vi "PLC_comm.vi"() -> ()   [LabVIEW 2017]
uses:
  <vilib>/addons/database/NI_Database_API.lvlib
  <vilib>/NI/Modbus Library/API/Wrapper/API Main.lvlib
  <vilib>/NI/Modbus Library/API/Wrapper/Create TCP Master.vi
  <vilib>/NI/Modbus Library/API/Master/Modbus Master.lvclass
  Global/DATA LOG.vi
  Global/Global 1.vi
  <vilib>/DATA AHEAD/SP7/typedefs/PLC Type.ctl
  <vilib>/DATA AHEAD/SP7/SP7.lvlib
  <vilib>/DATA AHEAD/SP7/functions/write/write bool array.vi
  <vilib>/DATA AHEAD/SP7/functions/read/read bool array.vi
  <vilib>/DATA AHEAD/SP7/functions/read/read int array.vi
  <vilib>/DATA AHEAD/SP7/functions/read/read String.vi
  <userlib>/_OpenG.lib/comparison/comparison.llb/String Changed__ogtk.vi
  <vilib>/addons/database/Connection.llb/DB Tools Open Connec (String).vi
panel:
  in  "timeout [ms]":i32=5000
  in  "String":string
  out "Array":u16[](array[numeric])
  out "element":u16
  out "length 2":i32
  out "substring":string
  out "length":i32
  out "reversed":string
  out "PLC 4":bool
  out "PLC 3":bool
  out "PLC 2":bool
  out "PLC 1":bool
  out "IP1 4":string
  out "IP1 3":string
  out "IP1 2":string
  out "IP1":string
  out "register values 4":u16[](array[numeric])
  out "ASCII VALUE 4":string[](array[string])
  out "BARCODE  4":string
  out "register values 3":u16[](array[numeric])
  out "ASCII VALUE 3":string[](array[string])
  out "BARCODE  3":string
  in  "stop":bool
  out "error out":errorcluster
  in  "error in (no error)":errorcluster
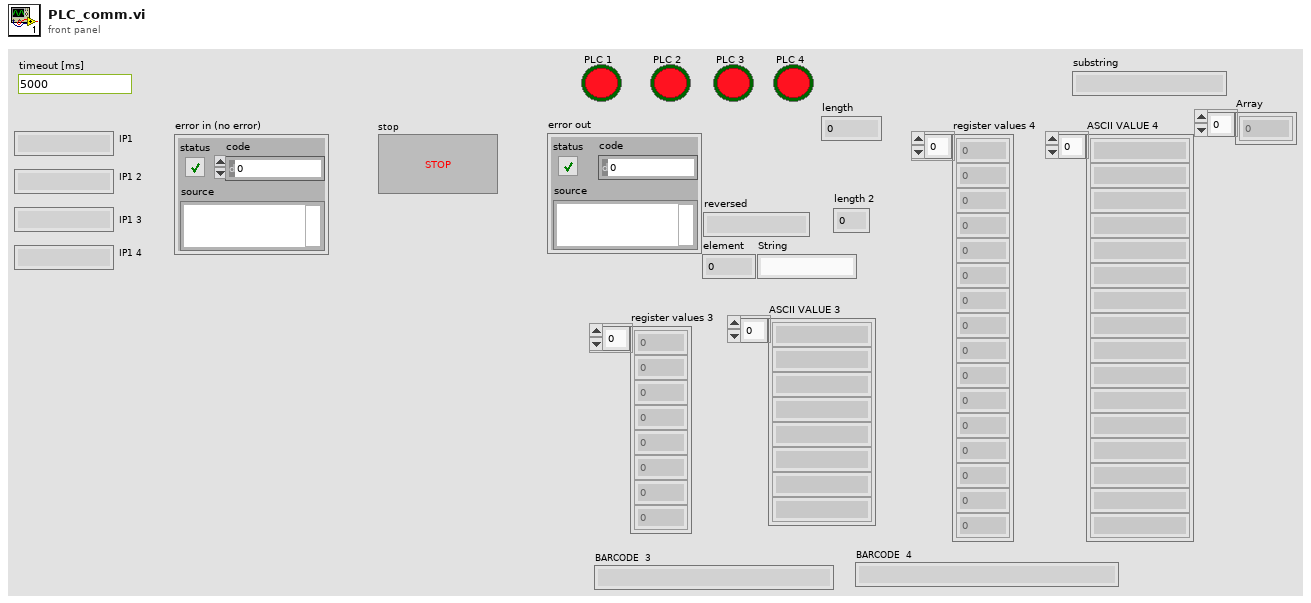
[diagram p1: front panel]
types:
  T1 = typedef "SP7.lvlib/PLC Type.ctl" = enum16{"S7 200", "S7 300/400", "S7 1200", "S7 1500", "LOGO!8"}
  T2 = typedef "NI_Database_API.lvlib/Conn ObjectReference.ctl" = refnum<k1>
  T3 = typedef "SP7.lvlib/S7 Connection.ctl" = cluster{"TCP Connection Ref":refnum<k5>, "IP address":string, "timeout ms":i32, "Connected?":bool, "PLC Type":T1, "Rack S7 400":u8, "Slot S7 400":u8, "PDU Size":u16, "connection semaphore":T4}
  T4 = typedef "Semaphore RefNum" = refnum<k1>
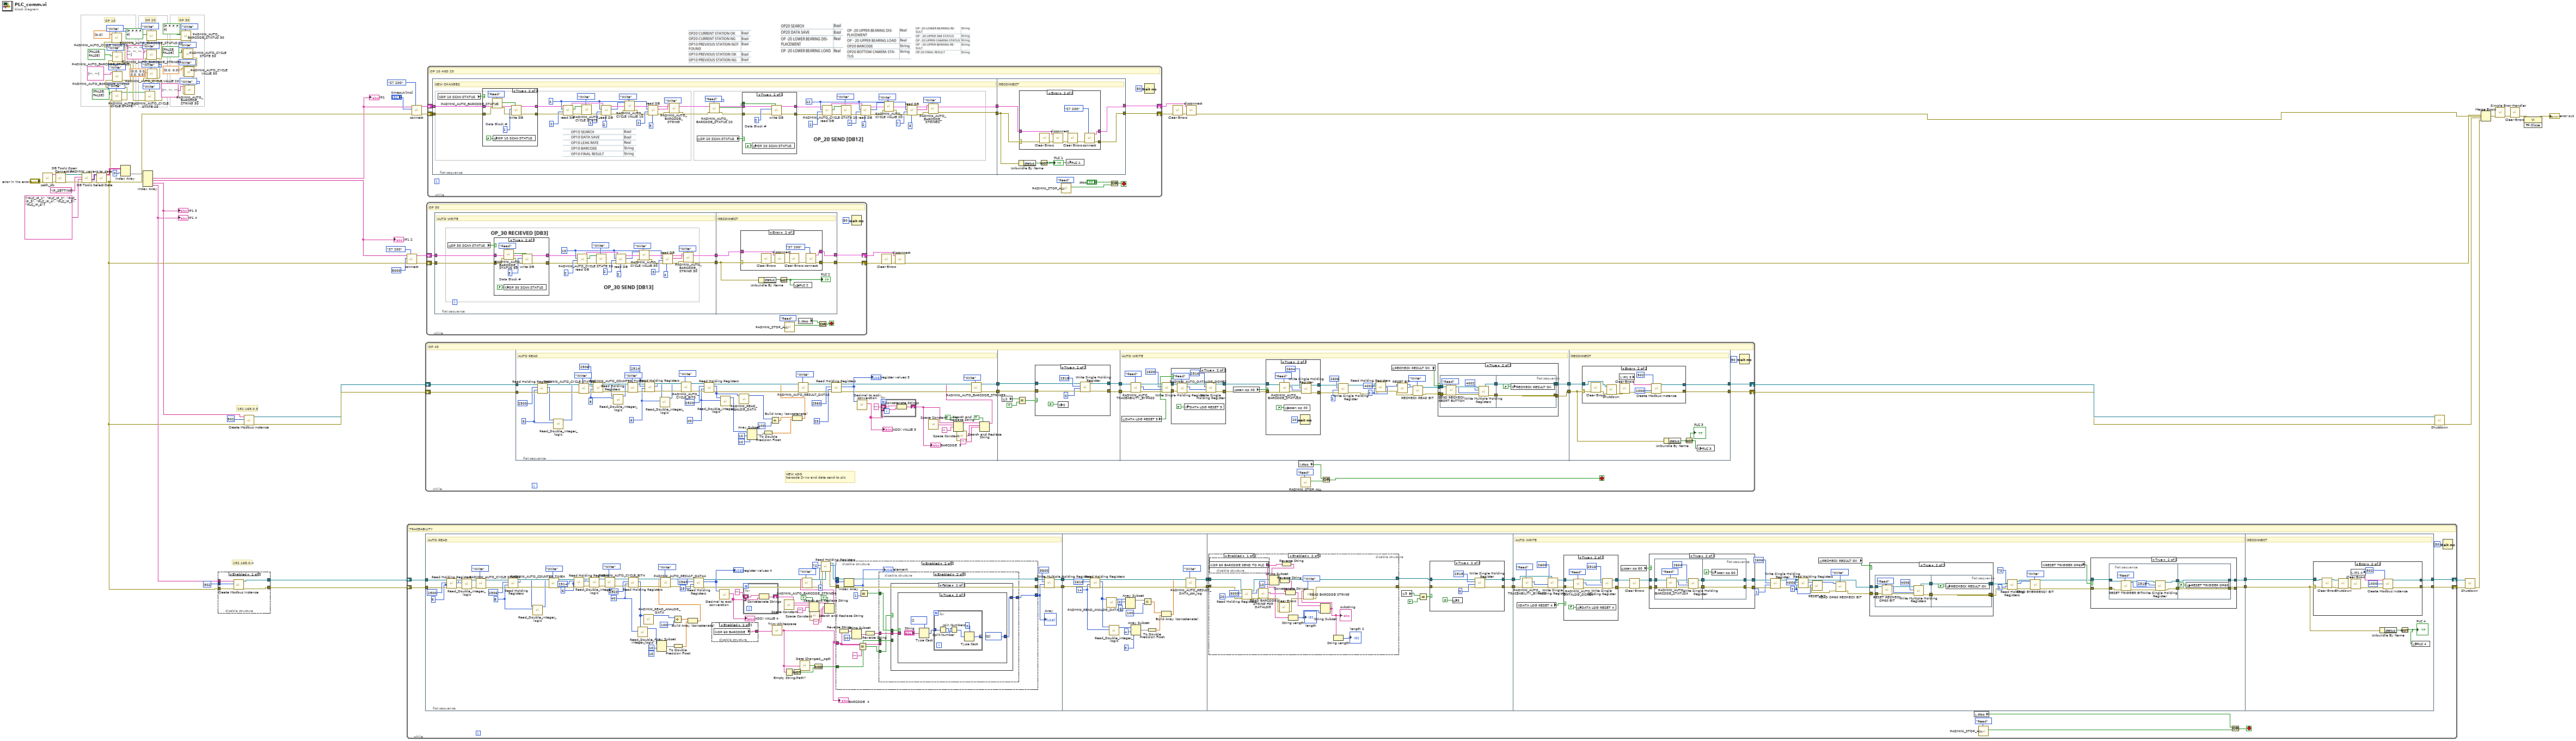
[diagram p0: block diagram]
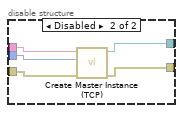
[diagram p2: hidden frame]
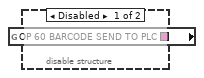
[diagram p3: hidden frame]
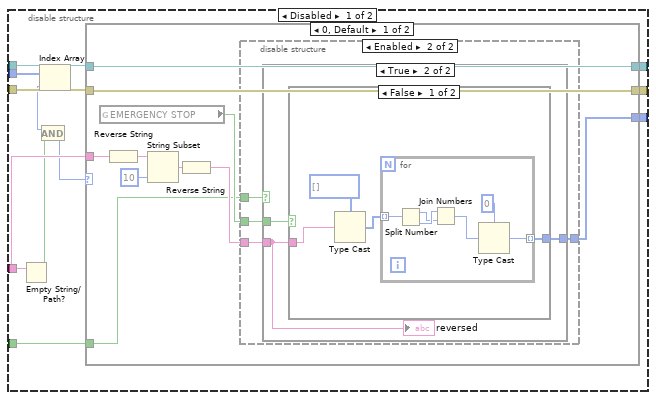
[diagram p4: hidden frame]
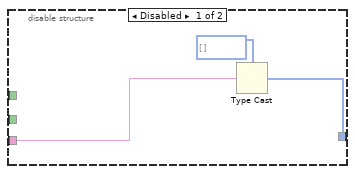
[diagram p5: hidden frame]
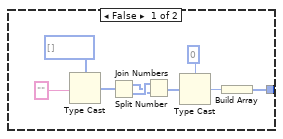
[diagram p6: hidden frame]
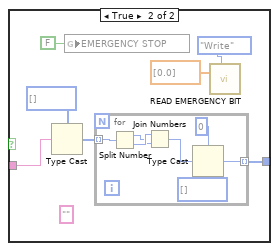
[diagram p7: hidden frame]
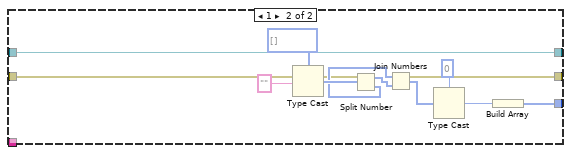
[diagram p8: hidden frame]
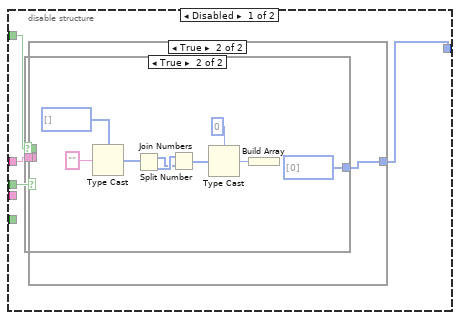
[diagram p9: hidden frame]
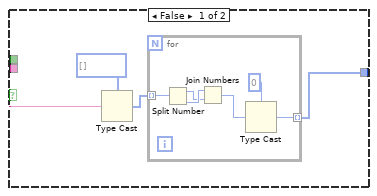
[diagram p10: hidden frame]
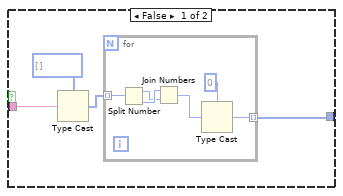
[diagram p11: hidden frame]
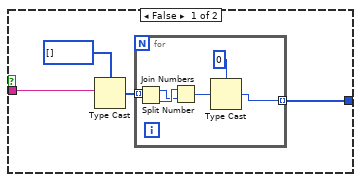
[diagram p12: hidden frame]
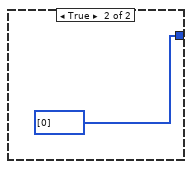
[diagram p13: hidden frame]
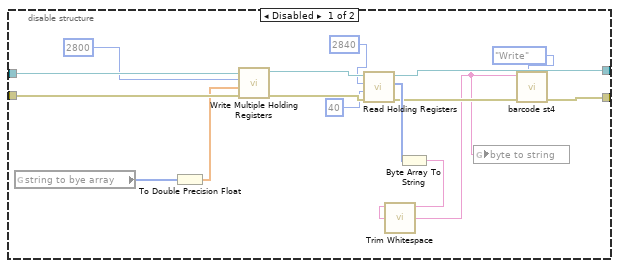
[diagram p14: hidden frame]
diagram:
  w31 = bool[] [FALSE, FALSE] ("Input")
  # "OP 30"
  # "OP 20"
  # "OP 10"
  # "192.168.0.3"
  # "192.168.0.4"
  n1 = call "path_db.vi"("error in"="error in (no error)") -> ("error out"=w78:errorcluster, "resulting string"=w83:string)  [unwired: 9 in]
  n2 = call-poly <vilib>:"DB Tools Open Connection.vi"("error in (no error)"=w78, "connection information"=w83) -> ("error out"=w82:errorcluster, "connection reference"=w81:T2)  [unwired: 6 in]
  n3 = call <vilib>:"DB Tools Select Data.vi"("error in (no error)"=w82, "columns"=string[] ["PLC_IP_1", "PLC_IP_2", "PLC_IP_3", "PLC_IP_4", "PLC_IP_5", "PLC_IP_6"], "table"="IP_SETTING", "connection reference"=w81) -> ("error out"=w80:errorcluster, "data"=w79:variant[][])  [unwired: 2 in, 1 out]
  n4 = call "PADMINI_varient_to_data.vi"("error in (no error)"=w80, "data"=w79) -> ("error out"=w46:errorcluster, "Array"=w74:string[][])  [unwired: 8 in]
  n5 = call "PADMINI_AUTO_CYCLE STATE.vi"("Enum"=enum16{"Read", "Write"}."Write", "error in (no error)"=w46, "Input"=w31) -> ("error out"=w44:errorcluster)  [unwired: 7 in, 1 out]
  n6 = call "PADMINI_AUTO_BARCODE_STRING.vi"("Enum"=enum16{"Read", "Write"}."Write", "error in (no error)"=w44, "Input"=string[] ["", ""]) -> ("error out"=w40:errorcluster)  [unwired: 7 in, 1 out]
  n7 = call "PADMINI_AUTO_BARCODE_STATUS.vi"("Enum"=enum16{"Read", "Write"}."Write", "error in (no error)"=w40, "I/P"=bool[] [FALSE, FALSE]) -> ("error out"=w38:errorcluster)  [unwired: 7 in, 1 out]
  n8 = call "PADMINI_AUTO_CYCLE VALUE 10.vi"("Enum"=enum16{"Read", "Write"}."Write", "error in (no error)"=w38, "Input"=dbl[] [0.0]) -> ("error out"=w32:errorcluster)  [unwired: 7 in, 1 out]
  n9 = Index Array(array=w74, index (row)=0) -> (element=w73:string[])  [unwired: 1 in]
  n10 = Index Array(array=w73) -> (element #1=w50:string, element #2=w17:string, element #3=w68:string, element #4=w67:string)  [unwired: 4 in]
  "IP1" <- w50
  "IP1 2" <- w17
  "IP1 3" <- w68
  "IP1 4" <- w67
  n11 = call "PADMINI_AUTO_CYCLE STATE 20.vi"("Enum"=enum16{"Read", "Write"}."Write", "error in (no error)"=w32, "Input"=w31) -> ("error out"=w29:errorcluster)  [unwired: 7 in, 1 out]
  n12 = call "PADMINI_AUTO_CYCLE VALUE 20.vi"("Enum"=enum16{"Read", "Write"}."Write", "error in (no error)"=w29, "Input"=dbl[] [0.0, 0.0, 0.0, 0.0]) -> ("error out"=w25:errorcluster)  [unwired: 7 in, 1 out]
  n13 = call "PADMINI_AUTO_BARCODE_STRING2.vi"("Enum"=enum16{"Read", "Write"}."Write", "error in (no error)"=w25, "Input"=string[] ["", "", "", "", "", "", ""]) -> ("error out"=w22:errorcluster)  [unwired: 7 in, 1 out]
  n14 = call "PADMINI_AUTO_BARCODE_STATUS 20.vi"("Enum"=enum16{"Read", "Write"}."Write", "error in (no error)"=w22, "I/P"=bool[] [FALSE, FALSE, FALSE, FALSE, FALSE]) -> ("error out"=w14:errorcluster)  [unwired: 7 in, 1 out]
  n15 = call "PADMINI_AUTO_BARCODE_STATUS 30.vi"("Enum"=enum16{"Read", "Write"}."Write", "error in (no error)"=w14, "I/P"=bool[] [FALSE, FALSE, FALSE, FALSE, FALSE]) -> ("error out"=w11:errorcluster)  [unwired: 7 in, 1 out]
  n16 = call "PADMINI_AUTO_CYCLE STATE 30.vi"("Enum"=enum16{"Read", "Write"}."Write", "error in (no error)"=w11, "Input"=bool[] [FALSE, FALSE]) -> ("error out"=w10:errorcluster)  [unwired: 7 in, 1 out]
  n17 = call "PADMINI_AUTO_CYCLE VALUE 30.vi"("Enum"=enum16{"Read", "Write"}."Write", "error in (no error)"=w10, "Input"=dbl[] [0.0, 0.0]) -> ("error out"=w6:errorcluster)  [unwired: 7 in, 1 out]
  n18 = call "PADMINI_AUTO_BARCODE_STRING 30.vi"("Enum"=enum16{"Read", "Write"}."Write", "error in (no error)"=w6, "Input"=string[] ["", "", ""]) -> ()  [unwired: 7 in, 2 out]
  n19 = disable-structure shown="Enabled" {
    disable-tunnel: w67 -> [w88 w92]
    disable-tunnel: u16 502 ("port (502)") -> [w87 w91]
    disable-tunnel: [w86 w90] -> w61
    disable-tunnel: [w85 w89] -> w60
    disable-tunnel: w46 -> [w84 w93]
    frame Enabled {
      n20 = call-poly <vilib>:"Create Modbus Instance.vi"("error in"=w84, "port (502)"=w87, "address"=w88) -> ("error out"=w85:errorcluster, "TCP master instance"=w86:refnum<class "Modbus Master.lvclass">)  [unwired: 7 in]
    }
    frame Disabled {
      n21 = call <vilib>:"Create Master Instance (TCP).vi"("error in (no error)"=w93, "port (502)"=w91, "address"=w92) -> ("error out"=w89:errorcluster, "TCP master instance"=w90:refnum<class "Modbus Master.lvclass">)  [unwired: 7 in]
    }
  }
  n22 = call-poly <vilib>:"Create Modbus Instance.vi"("error in"=w46, "port (502)"=u16 502, "address"=w68) -> ("error out"=w63:errorcluster, "TCP master instance"=w62:refnum<class "Modbus Master.lvclass">)  [unwired: 7 in]
  n23 = call <vilib>:"connect.vi"("PLC Type"=PLC_Type."S7 200" ("PLC Type 2"), "error in (no error)"=w46, "timeout [ms]"=5000 ("timeout [ms] 2"), "IP address"=w17) -> ("error out"=w19:errorcluster, "S7 Connection out"=w18:T3)  [unwired: 6 in]
  n24 = while {
    shift-right: [w108] -> w54
    shift-left: w61 -> [w110]
    shift-right: [w107] -> w55
    shift-left: w60 -> [w109]
    stop <- w101 stop-if-true
    # "TRACEABILITY"
    n25 = flat-sequence {
      tunnel: w110 -> [w183]
      tunnel: w109 -> [w182]
      tunnel: [w123] -> w100
      tunnel: [w126] -> w99
      tunnel: w100 -> [w352]
      tunnel: [w350] -> w98
      tunnel: w99 -> [w351]
      tunnel: [w348] -> w97
      tunnel: w98 -> [w370]
      tunnel: w97 -> [w368]
      tunnel: [w373] -> w96
      tunnel: [w372] -> w95
      tunnel: [w426] -> w105
      tunnel: w96 -> [w449]
      tunnel: w95 -> [w448]
      tunnel: [w424] -> w94
      tunnel: [w531] -> w107
      tunnel: [w533] -> w108
      tunnel: w105 -> [w534]
      tunnel: w94 -> [w529]
      frame #0 {
        (unwired) 10 ("length")
        w145 = u16 40 ("number of inputs")
        w147 = u16 6 ("number of inputs")
        w150 = u16 8 ("number of inputs")
        w153 = u16 6 ("number of inputs")
        # "AUTO READ"
        n26 = call-dynamic "Read Holding Registers.vi"("error in"=w182, "number of inputs"=w153, "starting address"=u16 2500, "Modbus master in"=w183) -> ("error out"=w175:errorcluster, "register values"=w154:u16[], "Modbus master out"=w174:refnum<class "Modbus Master.lvclass">)  [unwired: 5 in]
        n27 = call "Read_Double_integer_logic.vi"("Numeric"=w153, "register values"=w154) -> ("Array"=w152:u16[])  [unwired: 9 in]
        n28 = call "PADMINI_AUTO_CYCLE STATE4.vi"("Enum"=enum16{"Read", "Write"}."Write", "error in (no error)"=w175, "Input"=w152) -> ("error out"=w167:errorcluster)  [unwired: 7 in, 1 out]
        n29 = call-dynamic "Read Holding Registers.vi"("error in"=w167, "number of inputs"=w150, "starting address"=u16 2506, "Modbus master in"=w174) -> ("error out"=w173:errorcluster, "register values"=w151:u16[], "Modbus master out"=w172:refnum<class "Modbus Master.lvclass">)  [unwired: 5 in]
        n30 = call "Read_Double_integer_logic.vi"("Numeric"=w150, "register values"=w151) -> ("Array"=w149:u16[])  [unwired: 9 in]
        n31 = call "PADMINI_AUTO_COUNTER_TIME4.vi"("Enum"=enum16{"Read", "Write"}."Write", "error in (no error)"=w173, "Input"=w149) -> ("error out"=w165:errorcluster)  [unwired: 7 in, 1 out]
        n32 = call-dynamic "Read Holding Registers.vi"("error in"=w165, "number of inputs"=w147, "starting address"=u16 2514, "Modbus master in"=w172) -> ("error out"=w171:errorcluster, "register values"=w148:u16[], "Modbus master out"=w170:refnum<class "Modbus Master.lvclass">)  [unwired: 5 in]
        n33 = call "Read_Double_integer_logic.vi"("Numeric"=w147, "register values"=w148) -> ("Array"=w146:u16[])  [unwired: 9 in]
        n34 = call "PADMINI_AUTO_CYCLE_BIT4.vi"("Enum"=enum16{"Read", "Write"}."Write", "error in (no error)"=w171, "Input"=w146) -> ("error out"=w163:errorcluster)  [unwired: 7 in, 1 out]
        n35 = call-dynamic "Read Holding Registers.vi"("error in"=w163, "number of inputs"=w145, "starting address"=u16 2520, "Modbus master in"=w170) -> ("error out"=w169:errorcluster, "register values"=w142:u16[], "Modbus master out"=w168:refnum<class "Modbus Master.lvclass">)  [unwired: 5 in]
        n36 = call "Read_Double_integer_logic.vi"("Numeric"=w145, "register values"=w142) -> ("Array"=w144:u16[])  [unwired: 9 in]
        n37 = call "PADMINI_READ_ANALOG_DATA.vi"("register values"=w142) -> ("Array"=w141:i32[])  [unwired: 10 in]
        n38 = Array Subset(array=w144, index=10) -> (w157:u16[])  [unwired: 1 in]
        n39 = Divide(x=w141, y=u16 100 ("number of inputs")) -> (x/y=w155:dbl[])
        n40 = To Double Precision Float(number=w157) -> (double precision float=w156:dbl[])
        n41 = Build Array (concatenate)(w155, w156) -> (w143:dbl[])
        n42 = call "PADMINI_AUTO_RESULT_DATA4.vi"("Enum"=enum16{"Read", "Write"}."Write", "error in (no error)"=w169, "Input"=w143) -> ("error out"=w161:errorcluster)  [unwired: 7 in, 1 out]
        n43 = call-dynamic "Read Holding Registers.vi"("error in"=w161, "number of inputs"=u16 25, "starting address"=u16 2560, "Modbus master in"=w168) -> ("error out"=w121:errorcluster, "register values"=w176:u16[], "Modbus master out"=w119:refnum<class "Modbus Master.lvclass">)  [unwired: 5 in]
        "register values 4" <- w176
        n44 = disable-structure shown="Enabled" {
          disable-tunnel: [w187 w188] -> w120
          frame Disabled {
            n45 = global read "Global 1.vi" "OP 60 BARCODE SEND TO PLC"() -> (w187:string)
          }
          frame Enabled {
            n46 = global read "Global 1.vi" "OP 60 BARCODE"() -> (w188:string)
          }
        }
        n47 = call "Decimal to ascii converstion.vi"("DECIMAL VALUE"=w176) -> ("array w/ subset deleted"=w185:string[])  [unwired: 9 in]
        "ASCII VALUE 4" <- w185
        n48 = for {
          tunnel: w185 -> [w345] mode=indexing
          shift-right: [w344] -> w132
          shift-left: "" -> [w343]
          n49 = Concatenate Strings(w343, w345) -> (w344:string)
        }
        n50 = call <vilib>:"Trim Whitespace.vi"("string"=w120) -> ("trimmed string"=w111:string)  [unwired: 1 in]
        "BARCODE  4" <- w111
        n51 = call <vilib>:"Space Constant.vi"() -> ("String"=w140:string)
        n52 = Empty String/Path?(string/path=w111) -> (empty?=w129:bool)
        n53 = Not(x=w129) -> (.not. x?=w130:bool)
        n54 = call-poly <userlib>:"Data Changed__ogtk.vi"("String"=w111) -> ("Changed"=w128:bool)
        n55 = Search and Replace String(replace all?=TRUE ("replace all? (F)"), input string=w132, search string=w140, replace string="") -> (result string=w135:string)  [unwired: 4 in, 3 out]
        n56 = call <vilib>:"Space Constant.vi"() -> ("String"=w136:string)
        n57 = And(x=w128, y=w130) -> (x .and. y?=w112:bool)
        n58 = Search and Replace String(replace all?=TRUE ("replace all? (F)"), input string=w135, search string=w136, replace string="") -> (result string=w131:string)  [unwired: 4 in, 3 out]
        n59 = call "PADMINI_AUTO_BARCODE_STRING4.vi"("Enum"=enum16{"Read", "Write"}."Write", "error in (no error)"=w121, "Input"=w131) -> ("error out"=w118:errorcluster)  [unwired: 7 in, 1 out]
        n60 = call-dynamic "Read Holding Registers.vi"("error in"=w118, "number of inputs"=u16 3, "starting address"=u16 72, "Modbus master in"=w119) -> ("error out"=w116:errorcluster, "register values"=w113:u16[], "Modbus master out"=w117:refnum<class "Modbus Master.lvclass">)  [unwired: 5 in]
        n61 = disable-structure shown="Enabled" {
          disable-tunnel: w111 -> [w199 w265]
          disable-tunnel: w112 -> [w198 w274]
          disable-tunnel: [w197 w275] -> w127
          disable-tunnel: [w196 w276] -> w125
          disable-tunnel: [w195 w277] -> w124
          disable-tunnel: w117 -> [w194 w277]
          disable-tunnel: w116 -> [w193 w276]
          disable-tunnel: w113 -> [w192 w272]
          frame Disabled {
            n62 = Empty String/Path?(string/path=w199) -> (empty?=w190:bool)
            n63 = Index Array(array=w192) -> (element=w191:u16)  [unwired: 1 in]
            n64 = And(x=w191, y=w190) -> (x .and. y?=w189:u16)
            n65 = case shown="0, Default" w189 {
              tunnel: w194 -> [w201 w254]
              tunnel: [w201 w254] -> w195
              tunnel: w193 -> [w200 w253]
              tunnel: [w200 w253] -> w196
              tunnel: w199 -> [w205 _]
              tunnel: w198 -> [w203 _]
              tunnel: [w202 w252] -> w197
              frame 0, Default {
                n66 = global read "Global 1.vi" "EMERGENCY STOP"() -> (w204:bool)
                n67 = Reverse String(1:w205) -> (0:w209:string)
                n68 = String Subset(string=w209, length (rest)=10 ("length (rest)")) -> (substring=w207:string)  [unwired: 1 in]
                n69 = Reverse String(1:w207) -> (0:w206:string)
                n70 = disable-structure shown="Enabled" {
                  disable-tunnel: w206 -> [w212 w215]
                  disable-tunnel: [w211 w213] -> w202
                  disable-tunnel: w204 -> [_ w216]
                  disable-tunnel: w203 -> [_ w214]
                  frame Disabled {
                    n71 = Type Cast(type=u16[] [], x=w212) -> (*(type *) &x=w211:u16[])
                  }
                  frame Enabled {
                    n72 = case shown="True" w214 {
                      tunnel: w216 -> [_ w227]
                      tunnel: w215 -> [_ w226]
                      tunnel: [w217 w228] -> w213
                      frame False {
                        n73 = Type Cast(type=u16[] [], x="") -> (*(type *) &x=w224:u16[])
                        n74 = Split Number(x=w224) -> (hi(x)=w221:u8[], lo(x)=w222:u8[])
                        n75 = Join Numbers(hi=w222, lo=w221) -> ((hi.lo)=w220:u16[])
                        n76 = Type Cast(type=u16 0, x=w220) -> (*(type *) &x=w218:u16)
                        n77 = Build Array(w218) -> (w217:u16[])
                      }
                      frame True {
                        n78 = case shown="False" w227 {
                          tunnel: w226 -> [w230 w239]
                          tunnel: [w229 w242] -> w228
                          frame False {
                            n79 = Type Cast(type=u16[] [], x=w230) -> (*(type *) &x=w231:u16[])
                            n80 = for {
                              tunnel: w231 -> [w238] mode=indexing
                              tunnel: [w234] -> w229 mode=indexing
                              n81 = Split Number(x=w238) -> (hi(x)=w236:u8, lo(x)=w237:u8)
                              n82 = Join Numbers(hi=w237, lo=w236) -> ((hi.lo)=w235:u16)
                              n83 = Type Cast(type=u16 0, x=w235) -> (*(type *) &x=w234:u16)
                            }
                          }
                          frame True {
                            (unwired) ""
                            (unwired) u16[] []
                            n84 = Type Cast(type=u16[] [], x=w239) -> (*(type *) &x=w243:u16[])
                            n85 = global write "Global 1.vi" "EMERGENCY STOP"(FALSE ("EMERGENCY STOP")) -> ()
                            n86 = for {
                              tunnel: w243 -> [w251] mode=indexing
                              tunnel: [w247] -> w242 mode=indexing
                              n87 = Split Number(x=w251) -> (hi(x)=w249:u8, lo(x)=w250:u8)
                              n88 = Join Numbers(hi=w250, lo=w249) -> ((hi.lo)=w248:u16)
                              n89 = Type Cast(type=u16 0, x=w248) -> (*(type *) &x=w247:u16)
                            }
                            n90 = call "READ EMERGENCY BIT.vi"("Enum"=enum16{"Read", "Write"}."Write", "Array In"=dbl[] [0.0]) -> ()  [unwired: 8 in, 2 out]
                          }
                        }
                        "reversed" <- w226
                      }
                    }
                  }
                }
              }
              frame 1 {
                n91 = Type Cast(type=u16[] [], x="") -> (*(type *) &x=w261:u16[])
                n92 = Split Number(x=w261) -> (hi(x)=w258:u8[], lo(x)=w259:u8[])
                n93 = Join Numbers(hi=w259, lo=w258) -> ((hi.lo)=w257:u16[])
                n94 = Type Cast(type=u16 0, x=w257) -> (*(type *) &x=w255:u16)
                n95 = Build Array(w255) -> (w252:u16[])
              }
            }
          }
          frame Enabled {
            n96 = Reverse String(1:w265) -> (0:w270:string)
            n97 = Index Array(array=w272) -> (element=w273:u16)  [unwired: 1 in]
            "element" <- w273
            n98 = String Subset(string=w270, length (rest)=10 ("length (rest)")) -> (substring=w269:string)  [unwired: 1 in]
            n99 = Equal?(x=w265, y="") -> (x = y?=w263:bool)
            n100 = Equal?(x=w273, y=u16 1 ("x")) -> (x = y?=w266:bool)
            n101 = Reverse String(1:w269) -> (0:w267:string)
            n102 = disable-structure shown="Enabled" {
              disable-tunnel: [w281 w317] -> w275
              disable-tunnel: w274 -> [w280 w314]
              disable-tunnel: w266 -> [w279 w316]
              disable-tunnel: w267 -> [w278 w318]
              disable-tunnel: w265 -> [_ _]
              disable-tunnel: w263 -> [_ w315]
              frame Disabled {
                n103 = case shown="True" w280 {
                  tunnel: w278 -> [w283 w294]
                  tunnel: [w282 w293] -> w281
                  tunnel: w279 -> [_ w292]
                  frame False {
                    n104 = Type Cast(type=u16[] [], x=w283) -> (*(type *) &x=w284:u16[])
                    n105 = for {
                      tunnel: w284 -> [w291] mode=indexing
                      tunnel: [w287] -> w282 mode=indexing
                      n106 = Split Number(x=w291) -> (hi(x)=w289:u8, lo(x)=w290:u8)
                      n107 = Join Numbers(hi=w290, lo=w289) -> ((hi.lo)=w288:u16)
                      n108 = Type Cast(type=u16 0, x=w288) -> (*(type *) &x=w287:u16)
                    }
                  }
                  frame True {
                    n109 = case shown="True" w292 {
                      tunnel: w294 -> [w296 _]
                      tunnel: [w295 u16[] [0]] -> w293
                      frame False {
                        n110 = Type Cast(type=u16[] [], x=w296) -> (*(type *) &x=w297:u16[])
                        n111 = for {
                          tunnel: w297 -> [w304] mode=indexing
                          tunnel: [w300] -> w295 mode=indexing
                          n112 = Split Number(x=w304) -> (hi(x)=w302:u8, lo(x)=w303:u8)
                          n113 = Join Numbers(hi=w303, lo=w302) -> ((hi.lo)=w301:u16)
                          n114 = Type Cast(type=u16 0, x=w301) -> (*(type *) &x=w300:u16)
                        }
                      }
                      frame True {
                        n115 = Type Cast(type=u16[] [], x="" ("OP 60 BARCODE SEND TO PLC")) -> (*(type *) &x=w312:u16[])
                        n116 = Split Number(x=w312) -> (hi(x)=w309:u8[], lo(x)=w310:u8[])
                        n117 = Join Numbers(hi=w310, lo=w309) -> ((hi.lo)=w308:u16[])
                        n118 = Type Cast(type=u16 0, x=w308) -> (*(type *) &x=w306:u16)
                        n119 = Build Array(w306) -> ()  [unwired: 1 out]
                      }
                    }
                  }
                }
              }
              frame Enabled {
                n120 = case shown="False" w315 {
                  tunnel: w318 -> [w321 _]
                  tunnel: [w320 u16[] [0]] -> w317
                  tunnel: w316 -> [w319 _]
                  tunnel: w314 -> [_ _]
                  frame False {
                    n121 = case shown="True" w319 {
                      tunnel: w321 -> [w323 _]
                      tunnel: [w322 u16[] [0]] -> w320
                      frame False {
                        n122 = Type Cast(type=u16[] [], x=w323) -> (*(type *) &x=w324:u16[])
                        n123 = for {
                          tunnel: w324 -> [w331] mode=indexing
                          tunnel: [w326] -> w322 mode=indexing
                          n124 = Split Number(x=w331) -> (hi(x)=w329:u8, lo(x)=w330:u8)
                          n125 = Join Numbers(hi=w330, lo=w329) -> ((hi.lo)=w328:u16)
                          n126 = Type Cast(type=u16 0, x=w328) -> (*(type *) &x=w326:u16)
                        }
                      }
                      frame True {
                        n127 = Type Cast(type=u16[] [], x="String") -> (*(type *) &x=w334:u16[])
                        n128 = for {
                          tunnel: w334 -> [w341] mode=indexing
                          tunnel: [w337] -> _ mode=indexing
                          n129 = Split Number(x=w341) -> (hi(x)=w339:u8, lo(x)=w340:u8)
                          n130 = Join Numbers(hi=w340, lo=w339) -> ((hi.lo)=w338:u16)
                          n131 = Type Cast(type=u16 0, x=w338) -> (*(type *) &x=w337:u16)
                        }
                      }
                    }
                  }
                  frame True {
                  }
                }
              }
            }
          }
        }
        "Array" <- w127
        n132 = call-dynamic "Write Multiple Holding Registers.vi"("error in"=w125, "registers to write"=w127, "starting address"=u16 3600, "Modbus master in"=w124) -> ("error out"=w126:errorcluster, "Modbus master out"=w123:refnum<class "Modbus Master.lvclass">)  [unwired: 6 in]
      }
      frame #1 {
        w361 = u16 14 ("number of inputs")
        n133 = call-dynamic "Read Holding Registers.vi"("error in"=w351, "number of inputs"=w361, "starting address"=u16 2610, "Modbus master in"=w352) -> ("error out"=w349:errorcluster, "register values"=w359:u16[], "Modbus master out"=w350:refnum<class "Modbus Master.lvclass">)  [unwired: 5 in]
        n134 = call "PADMINI_READ_ANALOG_DATA 2y.vi"("register values"=w359) -> ("Array"=w354:i32[])  [unwired: 10 in]
        n135 = call "Read_Double_integer_logic.vi"("Numeric"=w361, "register values"=w359) -> ("Array"=w360:u16[])  [unwired: 9 in]
        n136 = Array Subset(array=w354, index=0, length=4) -> (w353:i32[])
        n137 = Array Subset(array=w360, index=4, length=3) -> (w364:u16[])
        n138 = Divide(x=w353, y=u16 100 ("number of inputs")) -> (x/y=w362:dbl[])
        n139 = To Double Precision Float(number=w364) -> (double precision float=w363:dbl[])
        n140 = Build Array (concatenate)(w362, w363) -> (w347:dbl[])
        n141 = call "PADMINI_AUTO_RESULT_DATA_st4_log.vi"("Enum"=enum16{"Read", "Write"}."Write", "error in (no error)"=w349, "Input"=w347) -> ("error out"=w348:errorcluster)  [unwired: 7 in, 1 out]
      }
      frame #2 {
        n142 = disable-structure shown="Enabled" {
          disable-tunnel: w370 -> [w390 w411]
          disable-tunnel: [w389 w410] -> w369
          disable-tunnel: w368 -> [w388 w409]
          disable-tunnel: [w387 w404] -> w367
          frame Disabled {
            n143 = global read "DATA LOG.vi" "string to bye array"() -> (w377:u8[])
            n144 = To Double Precision Float(number=w377) -> (double precision float=w376:dbl[])
            n145 = call-dynamic "Write Multiple Holding Registers.vi"("error in"=w388, "registers to write"=w376, "starting address"=u16 2800, "Modbus master in"=w390) -> ("error out"=w384:errorcluster, "Modbus master out"=w385:refnum<class "Modbus Master.lvclass">)  [unwired: 6 in]
            n146 = call-dynamic "Read Holding Registers.vi"("error in"=w384, "number of inputs"=u16 40 ("starting address"), "starting address"=u16 2840, "Modbus master in"=w385) -> ("error out"=w379:errorcluster, "register values"=w382:u16[], "Modbus master out"=w389:refnum<class "Modbus Master.lvclass">)  [unwired: 5 in]
            n147 = Byte Array To String(unsigned byte array=w382) -> (string=w378:string)
            n148 = call <vilib>:"Trim Whitespace.vi"("string"=w378) -> ()  [unwired: 1 in, 1 out]
            n149 = global write "DATA LOG.vi" "byte to string"(w378) -> ()
            n150 = call "barcode st4.vi"("Enum"=enum16{"Read", "Write"}."Write", "error in (no error)"=w379, "Input"=w378) -> ("error out"=w387:errorcluster)  [unwired: 7 in, 1 out]
          }
          frame Enabled {
            n151 = disable-structure shown="Enabled" {
              disable-tunnel: [w412 _] -> w397
              frame Enabled {
                n152 = global read "Global 1.vi" "OP 60 BARCODE SEND TO PLC"() -> (w412:string)
              }
              frame Disabled {
              }
            }
            n153 = call-dynamic "Read Holding Registers.vi"("error in"=w409, "number of inputs"=u16 20, "starting address"=u16 6000, "Modbus master in"=w411) -> ("error out"=w406:errorcluster, "register values"=w405:u16[], "Modbus master out"=w410:refnum<class "Modbus Master.lvclass">)  [unwired: 5 in]
            n154 = call "READ BARCODE STRING FOR DATALOG.vi"("error in (no error)"=w406, "DECIMAL VALUE"=w405) -> ("error out"=w392:errorcluster, "String"=w402:string)  [unwired: 7 in, 1 out]
            n155 = call <vilib>:"Clear Errors.vi"("error in (no error)"=w392) -> ("error out"=w391:errorcluster)  [unwired: 5 in, 1 out]
            n156 = Reverse String(1:w397) -> (0:w401:string)
            n157 = String Subset(string=w401, offset (0)=10) -> (substring=w399:string)  [unwired: 1 in]
            n158 = Reverse String(1:w399) -> (0:w398:string)
            n159 = Concatenate Strings(w398, w402) -> (w396:string)
            n160 = String Length(string=w397) -> (length=w395:i32)
            "length" <- w395
            n161 = String Subset(string=w396, length (rest)=w395) -> (substring=w393:string)  [unwired: 1 in]
            "substring" <- w393
            n162 = call "REAS BARCODE STRING.vi"("error in (no error)"=w391, "Input"=w393, "Enum"=enum16{"Read", "Write"}."Write") -> ("error out"=w404:errorcluster)  [unwired: 7 in, 1 out]
            n163 = String Length(string=w393) -> (length=→"length 2":i32)
          }
        }
        n164 = global read "DATA LOG.vi" "3"() -> (w375:bool)
        n165 = Equal?(x=w375, y=TRUE) -> (x = y?=w371:bool)
        n166 = case shown="True" w371 {
          tunnel: [w414 w419] -> w373
          tunnel: [w413 w418] -> w372
          tunnel: w369 -> [w414 w416]
          tunnel: w367 -> [w413 w415]
          frame False {
          }
          frame True {
            n167 = global write "DATA LOG.vi" "3"(FALSE) -> ()
            n168 = call-dynamic "Write Single Holding Register.vi"("error in"=w415, "register to write"=u16 0 ("address"), "address"=u16 2518, "Modbus master in"=w416) -> ("error out"=w418:errorcluster, "Modbus master out"=w419:refnum<class "Modbus Master.lvclass">)  [unwired: 6 in]
          }
        }
      }
      frame #3 {
        w443 = u16 2 ("number of inputs")
        # "AUTO WRITE"
        n169 = global read "DATA LOG.vi" "DATA LOG RESET 4"() -> (w452:bool)
        n170 = call "PADMINI_AUTO_TRACEABILITY_BYPASS.vi"("Enum"=enum16{"Read", "Write"}."Read", "error in (no error)"=w448) -> ("error out"=w460:errorcluster, "O/P"=w458:u16)  [unwired: 8 in]
        n171 = call-dynamic "Write Single Holding Register.vi"("error in"=w460, "register to write"=w458, "address"=u16 2600, "Modbus master in"=w449) -> ("error out"=w456:errorcluster, "Modbus master out"=w453:refnum<class "Modbus Master.lvclass">)  [unwired: 6 in]
        n172 = case shown="True" w452 {
          tunnel: w456 -> [w518 w528]
          tunnel: [w519 w527] -> w454
          tunnel: w453 -> [w519 w526]
          tunnel: [w518 w521] -> w423
          frame False {
          }
          frame True {
            n173 = call "PADMINI_AUTO_DATALOG_DONE4.vi"("Enum"=enum16{"Read", "Write"}."Read", "error in (no error)"=w528) -> ("error out"=w525:errorcluster, "O/P"=w522:u16)  [unwired: 8 in]
            n174 = global write "DATA LOG.vi" "DATA LOG RESET 4"(FALSE ("DATA LOG RESET 4")) -> ()
            n175 = call-dynamic "Write Single Holding Register.vi"("error in"=w525, "register to write"=w522, "address"=u16 2516, "Modbus master in"=w526) -> ("error out"=w521:errorcluster, "Modbus master out"=w527:refnum<class "Modbus Master.lvclass">)  [unwired: 6 in]
          }
        }
        n176 = global read "DATA LOG.vi" "scan op 60"() -> (w446:bool)
        n177 = call <vilib>:"Clear Errors.vi"("error in (no error)"=w423) -> ("error out"=w422:errorcluster)  [unwired: 5 in, 1 out]
        n178 = case shown="True" w446 {
          tunnel: [w500 w506] -> w455
          tunnel: w454 -> [w500 w505]
          tunnel: w422 -> [w499 w504]
          tunnel: [w499 w503] -> w451
          frame False {
          }
          frame True {
            n179 = flat-sequence {
              tunnel: w505 -> [w513]
              tunnel: w504 -> [w511]
              tunnel: [w514] -> w502
              tunnel: [w507] -> w501
              tunnel: [w516] -> w503
              tunnel: [w517] -> w506
              tunnel: w502 -> [w517]
              tunnel: w501 -> [w516]
              frame #0 {
                n180 = call "PADMINI_AUTO_BARCODE_STATUS4.vi"("Enum"=enum16{"Read", "Write"}."Read", "error in (no error)"=w511) -> ("error out"=w510:errorcluster, "O/P"=w509:u16)  [unwired: 8 in]
                n181 = call-dynamic "Write Single Holding Register.vi"("error in"=w510, "register to write"=w509, "address"=u16 2604, "Modbus master in"=w513) -> ("error out"=w507:errorcluster, "Modbus master out"=w514:refnum<class "Modbus Master.lvclass">)  [unwired: 6 in]
              }
              frame #1 {
                n182 = global write "DATA LOG.vi" "scan op 60"(FALSE ("scan op 60")) -> ()
              }
            }
          }
        }
        n183 = call-dynamic "Write Single Holding Register.vi"("error in"=w451, "register to write"=u16 1 ("address"), "address"=u16 2606, "Modbus master in"=w455) -> ("error out"=w440:errorcluster, "Modbus master out"=w437:refnum<class "Modbus Master.lvclass">)  [unwired: 6 in]
        n184 = call-dynamic "Read Holding Registers.vi"("error in"=w440, "number of inputs"=w443, "starting address"=u16 4006, "Modbus master in"=w437) -> ("error out"=w445:errorcluster, "register values"=w444:u16[])  [unwired: 5 in, 1 out]
        n185 = call "RESET BIT.vi"("Numeric"=w443, "register values"=w444) -> ("Array"=w439:u16[])  [unwired: 9 in]
        n186 = global read "Global 1.vi" "RECHECK RESULT OK"() -> (w438:bool)
        n187 = call "READ OP60 RECHECK BIT.vi"("Enum"=enum16{"Read", "Write"}."Write", "error in (no error)"=w445, "Input"=w439) -> ("error out"=w436:errorcluster)  [unwired: 7 in, 1 out]
        n188 = case shown="True" w438 {
          tunnel: w437 -> [w481 w482]
          tunnel: [w481 w487] -> w434
          tunnel: w436 -> [w480 w486]
          tunnel: [w480 w485] -> w431
          frame False {
          }
          frame True {
            n189 = flat-sequence {
              tunnel: w486 -> [w490]
              tunnel: [w494] -> w484
              tunnel: [w489] -> w483
              tunnel: w482 -> [w488]
              tunnel: [w497] -> w485
              tunnel: [w498] -> w487
              tunnel: w484 -> [w498]
              tunnel: w483 -> [w497]
              frame #0 {
                n190 = call "RESET RECHECK OP60 BIT.vi"("Enum"=enum16{"Read", "Write"}."Read", "error in (no error)"=w490) -> ("error out"=w491:errorcluster, "Array 2"=w493:u16[])  [unwired: 8 in]
                n191 = call-dynamic "Write Multiple Holding Registers.vi"("error in"=w491, "registers to write"=w493, "starting address"=u16 4006, "Modbus master in"=w488) -> ("error out"=w489:errorcluster, "Modbus master out"=w494:refnum<class "Modbus Master.lvclass">)  [unwired: 6 in]
              }
              frame #1 {
                n192 = global write "Global 1.vi" "RECHECK RESULT OK"(FALSE ("RECHECK RESULT OK")) -> ()
              }
            }
          }
        }
        n193 = call-dynamic "Read Holding Registers.vi"("error in"=w431, "number of inputs"=u16 1, "starting address"=u16 70 ("address"), "Modbus master in"=w434) -> ("error out"=w430:errorcluster, "register values"=w429:u16[], "Modbus master out"=w427:refnum<class "Modbus Master.lvclass">)  [unwired: 5 in]
        n194 = call "READ EMERGENCY BIT.vi"("Enum"=enum16{"Read", "Write"}."Write", "error in (no error)"=w430, "Array In"=w429) -> ("error out"=w425:errorcluster)  [unwired: 7 in, 1 out]
        n195 = global read "Global 1.vi" "RESET TRIGGER OP60"() -> (w428:bool)
        n196 = case shown="True" w428 {
          tunnel: w427 -> [w462 w468]
          tunnel: w425 -> [w461 w467]
          tunnel: [w462 w466] -> w426
          tunnel: [w461 w464] -> w424
          frame False {
          }
          frame True {
            n197 = flat-sequence {
              tunnel: w468 -> [w476]
              tunnel: w467 -> [w472]
              tunnel: [w475] -> w465
              tunnel: [w474] -> w463
              tunnel: [w479] -> w466
              tunnel: w465 -> [w479]
              tunnel: [w478] -> w464
              tunnel: w463 -> [w478]
              frame #0 {
                n198 = call "RESET TRIGGER BIT.vi"("Enum"=enum16{"Read", "Write"}."Read", "error in (no error)"=w472) -> ("error out"=w471:errorcluster, "Numeric 2"=w469:u16)  [unwired: 8 in]
                n199 = call-dynamic "Write Single Holding Register.vi"("error in"=w471, "register to write"=w469, "address"=u16 2518 ("starting address"), "Modbus master in"=w476) -> ("error out"=w474:errorcluster, "Modbus master out"=w475:refnum<class "Modbus Master.lvclass">)  [unwired: 6 in]
              }
              frame #1 {
                n200 = global write "Global 1.vi" "RESET TRIGGER OP60"(FALSE ("RESET TRIGGER OP60")) -> ()
              }
            }
          }
        }
      }
      frame #4 {
        # "RECONNECT"
        n201 = case shown="Error" w529 {
          selector: w529 -> [w535 w545]
          tunnel: [w536 w542] -> w533
          tunnel: w534 -> [w536 w540]
          tunnel: [w535 w541] -> w531
          frame No Error {
          }
          frame Error {
            n202 = call <vilib>:"Clear Errors.vi"("error in (no error)"=w545) -> ("error out"=w539:errorcluster)  [unwired: 5 in, 1 out]
            n203 = call-dynamic "Shutdown.vi"("error in"=w539, "Modbus master in"=w540) -> ("error out"=w538:errorcluster)  [unwired: 9 in]
            n204 = local read "IP1 4"() -> (w543:string)
            n205 = call <vilib>:"Clear Errors.vi"("error in (no error)"=w538) -> ("error out"=w544:errorcluster)  [unwired: 5 in, 1 out]
            n206 = call-poly <vilib>:"Create Modbus Instance.vi"("error in"=w544, "connect timeout ms"=1000, "port (502)"=u16 502, "address"=w543) -> ("error out"=w541:errorcluster, "TCP master instance"=w542:refnum<class "Modbus Master.lvclass">)  [unwired: 6 in]
          }
        }
        n207 = Unbundle By Name(w529) -> ("status"=w532:bool)
        n208 = Not(x=w532) -> (.not. x?=w530:bool)
        "PLC 4" <- w530
        n209 = global write "Global 1.vi" "PLC 4"(w530) -> ()
      }
    }
    n210 = local read "stop"() -> (w102:bool)
    n211 = call "PADMINI_STOP_ALL.vi"("Enum"=enum16{"Read", "Write"}."Read") -> ("Boolean 2"=w103:bool)  [unwired: 9 in, 1 out]
    n212 = Or(x=w102, y=w103) -> (x .or. y?=w101:bool)
    n213 = Wait (ms)(milliseconds to wait=u32 50) -> ()  [unwired: 1 out]
  }
  n214 = call <vilib>:"connect.vi"("PLC Type"=PLC_Type."S7 200" ("PLC Type 2"), "error in (no error)"=w46, "timeout [ms]"="timeout [ms]", "IP address"=w50) -> ("error out"=w49:errorcluster, "S7 Connection out"=w48:T3)  [unwired: 6 in]
  n215 = while {
    shift-right: [w559] -> w58
    shift-left: w62 -> [w561]
    shift-right: [w558] -> w57
    shift-left: w63 -> [w560]
    stop <- w551 stop-if-true
    # "NEW ADD\nbarcode Sr no and date send to plc"
    # "OP 40"
    n216 = flat-sequence {
      tunnel: w561 -> [w618]
      tunnel: w560 -> [w617]
      tunnel: [w603] -> w550
      tunnel: [w594] -> w548
      tunnel: w550 -> [w628]
      tunnel: [w629] -> w549
      tunnel: w548 -> [w627]
      tunnel: [w626] -> w547
      tunnel: w549 -> [w665]
      tunnel: [w644] -> w556
      tunnel: [w642] -> w555
      tunnel: w547 -> [w669]
      tunnel: [w714] -> w558
      tunnel: [w717] -> w559
      tunnel: w556 -> [w716]
      tunnel: w555 -> [w712]
      frame #0 {
        w581 = u16 40 ("number of inputs")
        w585 = u16 6 ("number of inputs")
        w588 = u16 8 ("number of inputs")
        w589 = u16 6 ("number of inputs")
        # "AUTO READ"
        n217 = call-dynamic "Read Holding Registers.vi"("error in"=w617, "number of inputs"=w589, "starting address"=u16 2500, "Modbus master in"=w618) -> ("error out"=w611:errorcluster, "register values"=w592:u16[], "Modbus master out"=w610:refnum<class "Modbus Master.lvclass">)  [unwired: 5 in]
        n218 = call "Read_Double_integer_logic.vi"("Numeric"=w589, "register values"=w592) -> ("Array"=w590:u16[])  [unwired: 9 in]
        n219 = call "PADMINI_AUTO_CYCLE STATE3.vi"("Enum"=enum16{"Read", "Write"}."Write", "error in (no error)"=w611, "Input"=w590) -> ("error out"=w602:errorcluster)  [unwired: 7 in, 1 out]
        n220 = call-dynamic "Read Holding Registers.vi"("error in"=w602, "number of inputs"=w588, "starting address"=u16 2506, "Modbus master in"=w610) -> ("error out"=w609:errorcluster, "register values"=w587:u16[], "Modbus master out"=w608:refnum<class "Modbus Master.lvclass">)  [unwired: 5 in]
        n221 = call "Read_Double_integer_logic.vi"("Numeric"=w588, "register values"=w587) -> ("Array"=w586:u16[])  [unwired: 9 in]
        n222 = call "PADMINI_AUTO_COUNTER_TIME3.vi"("Enum"=enum16{"Read", "Write"}."Write", "error in (no error)"=w609, "Input"=w586) -> ("error out"=w600:errorcluster)  [unwired: 7 in, 1 out]
        n223 = call-dynamic "Read Holding Registers.vi"("error in"=w600, "number of inputs"=w585, "starting address"=u16 2514, "Modbus master in"=w608) -> ("error out"=w607:errorcluster, "register values"=w584:u16[], "Modbus master out"=w606:refnum<class "Modbus Master.lvclass">)  [unwired: 5 in]
        n224 = call "Read_Double_integer_logic.vi"("Numeric"=w585, "register values"=w584) -> ("Array"=w583:u16[])  [unwired: 9 in]
        n225 = call "PADMINI_AUTO_CYCLE_BIT3.vi"("Enum"=enum16{"Read", "Write"}."Write", "error in (no error)"=w607, "Input"=w583) -> ("error out"=w598:errorcluster)  [unwired: 7 in, 1 out]
        n226 = call-dynamic "Read Holding Registers.vi"("error in"=w598, "number of inputs"=w581, "starting address"=u16 2520, "Modbus master in"=w606) -> ("error out"=w605:errorcluster, "register values"=w572:u16[], "Modbus master out"=w582:refnum<class "Modbus Master.lvclass">)  [unwired: 5 in]
        n227 = call "Read_Double_integer_logic.vi"("Numeric"=w581, "register values"=w572) -> ("Array"=w577:u16[])  [unwired: 9 in]
        n228 = call "PADMINI_READ_ANALOG_DATA.vi"("register values"=w572) -> ("Array"=w571:i32[])  [unwired: 10 in]
        n229 = Array Subset(array=w577, index=10, length=10) -> (w576:u16[])
        n230 = To Double Precision Float(number=w576) -> (double precision float=w575:dbl[])
        n231 = Divide(x=w571, y=u16 100 ("number of inputs")) -> (x/y=w574:dbl[])
        n232 = Build Array (concatenate)(w574, w575) -> (w573:dbl[])
        n233 = call "PADMINI_AUTO_RESULT_DATA3.vi"("Enum"=enum16{"Read", "Write"}."Write", "error in (no error)"=w605, "Input"=w573) -> ("error out"=w596:errorcluster)  [unwired: 7 in, 1 out]
        n234 = call-dynamic "Read Holding Registers.vi"("error in"=w596, "number of inputs"=u16 25, "starting address"=u16 2560, "Modbus master in"=w582) -> ("error out"=w604:errorcluster, "register values"=w612:u16[], "Modbus master out"=w603:refnum<class "Modbus Master.lvclass">)  [unwired: 5 in]
        "register values 3" <- w612
        n235 = call "Decimal to ascii converstion.vi"("DECIMAL VALUE"=w612) -> ("array w/ subset deleted"=w620:string[])  [unwired: 9 in]
        "ASCII VALUE 3" <- w620
        n236 = for {
          tunnel: w620 -> [w624] mode=indexing
          shift-right: [w623] -> w563
          shift-left: "" -> [w622]
          n237 = Concatenate Strings(w622, w624) -> (w623:string)
        }
        "BARCODE  3" <- w563
        n238 = call <vilib>:"Space Constant.vi"() -> ("String"=w570:string)
        n239 = Search and Replace String(replace all?=TRUE ("replace all? (F)"), input string=w563, search string=w570, replace string="") -> (result string=w565:string)  [unwired: 4 in, 3 out]
        n240 = call <vilib>:"Space Constant.vi"() -> ("String"=w566:string)
        n241 = Search and Replace String(replace all?=TRUE ("replace all? (F)"), input string=w565, search string=w566, replace string="") -> (result string=w562:string)  [unwired: 4 in, 3 out]
        n242 = call "PADMINI_AUTO_BARCODE_STRING3.vi"("Enum"=enum16{"Read", "Write"}."Write", "error in (no error)"=w604, "Input"=w562) -> ("error out"=w594:errorcluster)  [unwired: 7 in, 1 out]
      }
      frame #1 {
        n243 = global read "DATA LOG.vi" "2"() -> (w630:bool)
        n244 = Equal?(x=w630, y=TRUE) -> (x = y?=w625:bool)
        n245 = case shown="True" w625 {
          tunnel: w628 -> [w632 w638]
          tunnel: w627 -> [w633 w636]
          tunnel: [w632 w637] -> w629
          tunnel: [w633 w635] -> w626
          frame False {
          }
          frame True {
            n246 = global write "DATA LOG.vi" "2"(FALSE) -> ()
            n247 = call-dynamic "Write Single Holding Register.vi"("error in"=w636, "register to write"=u16 0 ("address"), "address"=u16 2518, "Modbus master in"=w638) -> ("error out"=w635:errorcluster, "Modbus master out"=w637:refnum<class "Modbus Master.lvclass">)  [unwired: 6 in]
          }
        }
      }
      frame #2 {
        w651 = u16 2 ("number of inputs")
        # "AUTO WRITE"
        n248 = global read "DATA LOG.vi" "DATA LOG RESET 3"() -> (w657:bool)
        n249 = call "PADMINI_AUTO_TRACEABILITY_BYPASS.vi"("Enum"=enum16{"Read", "Write"}."Read", "error in (no error)"=w669) -> ("error out"=w668:errorcluster, "O/P"=w666:u16)  [unwired: 8 in]
        n250 = call-dynamic "Write Single Holding Register.vi"("error in"=w668, "register to write"=w666, "address"=u16 2600, "Modbus master in"=w665) -> ("error out"=w663:errorcluster, "Modbus master out"=w660:refnum<class "Modbus Master.lvclass">)  [unwired: 6 in]
        n251 = case shown="True" w657 {
          tunnel: w663 -> [w702 w711]
          tunnel: [w701 w710] -> w661
          tunnel: w660 -> [w701 w709]
          tunnel: [w702 w704] -> w658
          frame False {
          }
          frame True {
            n252 = call "PADMINI_AUTO_DATALOG_DONE3.vi"("Enum"=enum16{"Read", "Write"}."Read", "error in (no error)"=w711) -> ("error out"=w708:errorcluster, "O/P"=w705:u16)  [unwired: 8 in]
            n253 = global write "DATA LOG.vi" "DATA LOG RESET 3"(FALSE ("DATA LOG RESET 3")) -> ()
            n254 = call-dynamic "Write Single Holding Register.vi"("error in"=w708, "register to write"=w705, "address"=u16 2516, "Modbus master in"=w709) -> ("error out"=w704:errorcluster, "Modbus master out"=w710:refnum<class "Modbus Master.lvclass">)  [unwired: 6 in]
          }
        }
        n255 = global read "DATA LOG.vi" "scan op 40"() -> (w654:bool)
        n256 = case shown="True" w654 {
          tunnel: [w690 w700] -> w662
          tunnel: w661 -> [w690 w699]
          tunnel: w658 -> [w689 w698]
          tunnel: [w689 w697] -> w656
          frame False {
          }
          frame True {
            n257 = call "PADMINI_AUTO_BARCODE_STATUS3.vi"("Enum"=enum16{"Read", "Write"}."Read", "error in (no error)"=w698) -> ("error out"=w695:errorcluster, "O/P"=w694:u16)  [unwired: 8 in]
            n258 = global write "DATA LOG.vi" "scan op 40"(FALSE ("scan op 40")) -> ()
            n259 = Wait (ms)(milliseconds to wait=u32 20) -> ()  [unwired: 1 out]
            n260 = call-dynamic "Write Single Holding Register.vi"("error in"=w695, "register to write"=w694, "address"=u16 2604, "Modbus master in"=w699) -> ("error out"=w697:errorcluster, "Modbus master out"=w700:refnum<class "Modbus Master.lvclass">)  [unwired: 6 in]
          }
        }
        n261 = call-dynamic "Write Single Holding Register.vi"("error in"=w656, "register to write"=u16 1 ("address"), "address"=u16 2606, "Modbus master in"=w662) -> ("error out"=w646:errorcluster, "Modbus master out"=w648:refnum<class "Modbus Master.lvclass">)  [unwired: 6 in]
        n262 = call-dynamic "Read Holding Registers.vi"("error in"=w646, "number of inputs"=w651, "starting address"=u16 4002, "Modbus master in"=w648) -> ("error out"=w647:errorcluster, "register values"=w653:u16[], "Modbus master out"=w645:refnum<class "Modbus Master.lvclass">)  [unwired: 5 in]
        n263 = global read "Global 1.vi" "RECHECK RESULT OK"() -> (w641:bool)
        n264 = call "RESET BIT.vi"("Numeric"=w651, "register values"=w653) -> ("Array"=w652:u16[])  [unwired: 9 in]
        n265 = call "RECHECK READ BIT.vi"("Enum"=enum16{"Read", "Write"}."Write", "error in (no error)"=w647, "Input"=w652) -> ("error out"=w643:errorcluster)  [unwired: 7 in, 1 out]
        n266 = case shown="True" w641 {
          tunnel: w645 -> [w671 w677]
          tunnel: [w671 w676] -> w644
          tunnel: w643 -> [w670 w675]
          tunnel: [w670 w674] -> w642
          frame False {
          }
          frame True {
            n267 = flat-sequence {
              tunnel: w677 -> [w684]
              tunnel: w675 -> [w679]
              tunnel: [w683] -> w673
              tunnel: [w678] -> w672
              tunnel: [w687] -> w674
              tunnel: [w688] -> w676
              tunnel: w673 -> [w688]
              tunnel: w672 -> [w687]
              frame #0 {
                n268 = call "SEND RECHECK ABORT BUTTON.vi"("Enum"=enum16{"Read", "Write"}."Read", "error in (no error)"=w679) -> ("error out"=w680:errorcluster, "Array 2"=w682:u16[])  [unwired: 8 in]
                n269 = call-dynamic "Write Multiple Holding Registers.vi"("error in"=w680, "registers to write"=w682, "starting address"=u16 4002, "Modbus master in"=w684) -> ("error out"=w678:errorcluster, "Modbus master out"=w683:refnum<class "Modbus Master.lvclass">)  [unwired: 6 in]
              }
              frame #1 {
                n270 = global write "Global 1.vi" "RECHECK RESULT OK"(FALSE ("RECHECK RESULT OK")) -> ()
              }
            }
          }
        }
      }
      frame #3 {
        # "RECONNECT"
        n271 = case shown="Error" w712 {
          selector: w712 -> [w718 w728]
          tunnel: [w719 w725] -> w717
          tunnel: w716 -> [w719 w721]
          tunnel: [w718 w724] -> w714
          frame No Error {
          }
          frame Error {
            n272 = call <vilib>:"Clear Errors.vi"("error in (no error)"=w728) -> ("error out"=w723:errorcluster)  [unwired: 5 in, 1 out]
            n273 = call-dynamic "Shutdown.vi"("error in"=w723, "Modbus master in"=w721) -> ("error out"=w722:errorcluster)  [unwired: 9 in]
            n274 = local read "IP1 3"() -> (w726:string)
            n275 = call <vilib>:"Clear Errors.vi"("error in (no error)"=w722) -> ("error out"=w727:errorcluster)  [unwired: 5 in, 1 out]
            n276 = call-poly <vilib>:"Create Modbus Instance.vi"("error in"=w727, "connect timeout ms"=1000, "port (502)"=u16 502, "address"=w726) -> ("error out"=w724:errorcluster, "TCP master instance"=w725:refnum<class "Modbus Master.lvclass">)  [unwired: 6 in]
          }
        }
        n277 = Unbundle By Name(w712) -> ("status"=w715:bool)
        n278 = Not(x=w715) -> (.not. x?=w713:bool)
        "PLC 3" <- w713
        n279 = global write "Global 1.vi" "PLC 3"(w713) -> ()
      }
    }
    n280 = local read "stop"() -> (w552:bool)
    n281 = call "PADMINI_STOP_ALL.vi"("Enum"=enum16{"Read", "Write"}."Read") -> ("Boolean 2"=w553:bool)  [unwired: 9 in, 1 out]
    n282 = Or(x=w552, y=w553) -> (x .or. y?=w551:bool)
    n283 = Wait (ms)(milliseconds to wait=u32 50) -> ()  [unwired: 1 out]
  }
  n284 = while {
    shift-right: [w730] -> w3
    shift-left: w18 -> [w740]
    shift-right: [w738] -> w2
    shift-left: w19 -> [w739]
    stop <- w732 stop-if-true
    # "OP 30"
    n285 = flat-sequence {
      tunnel: [w742] -> w736
      tunnel: [w741] -> w731
      tunnel: w739 -> [w766]
      tunnel: w740 -> [w765]
      tunnel: [w779] -> w738
      tunnel: [w778] -> w730
      tunnel: w736 -> [w781]
      tunnel: w731 -> [w780]
      frame #0 {
        w755 = u16 13 ("Data Block #")
        # "AUTO WRITE"
        n286 = global read "DATA LOG.vi" "OP 30 SCAN STATUS"() -> (w764:bool)
        n287 = case shown="True" w764 {
          tunnel: w765 -> [w767 w776]
          tunnel: [w768 w775] -> w743
          tunnel: [w767 w774] -> w744
          tunnel: w766 -> [w768 w771]
          frame False {
          }
          frame True {
            w777 = u16 3  # Data Block #
            n288 = call "PADMINI_AUTO_BARCODE_STATUS 30.vi"("Enum"=enum16{"Read", "Write"}."Read", "error in (no error)"=w771) -> ("error out"=w770:errorcluster, "O/P"=w772:bool[])  [unwired: 8 in]
            n289 = global write "DATA LOG.vi" "OP 30 SCAN STATUS"(FALSE) -> ()
            n290 = call-poly <vilib>:"write DB.vi"("BOOL input array [byte]"=w772, "error in (no error)"=w770, "Data Block #"=w777, "S7 Connection in"=w776) -> ("error out"=w775:errorcluster, "S7 Connection out"=w774:T3)  [unwired: 4 in, 2 out]
          }
        }
        n291 = call-poly <vilib>:"read DB.vi"("error in (no error)"=w743, "Items # [byte]"=u16 2, "Data Block #"=w755, "S7 Connection in"=w744) -> ("error out"=w762:errorcluster, "BOOL result array  [byte]"=w760:bool[], "S7 Connection out"=w757:T3)  [unwired: 5 in]
        n292 = call "PADMINI_AUTO_CYCLE STATE 30.vi"("Enum"=enum16{"Read", "Write"}."Write", "error in (no error)"=w762, "Input"=w760) -> ("error out"=w758:errorcluster)  [unwired: 7 in, 1 out]
        n293 = call-poly <vilib>:"read DB.vi"("Item offset [byte]"=u32 2, "error in (no error)"=w758, "items #"=u16 2 ("Items # [byte]"), "Data Block #"=w755, "S7 Connection in"=w757) -> ("error out"=w747:errorcluster, "Int result array"=w745:i16[], "S7 Connection out"=w756:T3)  [unwired: 4 in]
        n294 = call "PADMINI_AUTO_CYCLE VALUE 30.vi"("Enum"=enum16{"Read", "Write"}."Write", "error in (no error)"=w747, "Input"=w745) -> ("error out"=w746:errorcluster)  [unwired: 7 in, 1 out]
        n295 = call-poly <vilib>:"read DB.vi"("Item offset [byte]"=u32 4, "error in (no error)"=w746, "items #"=u16 3 ("Items # [byte]"), "Data Block #"=w755, "S7 Connection in"=w756) -> ("error out"=w751:errorcluster, "STRING result Array"=w752:string[], "S7 Connection out"=w742:T3)  [unwired: 3 in, 1 out]
        n296 = call "PADMINI_AUTO_BARCODE_STRING 30.vi"("Enum"=enum16{"Read", "Write"}."Write", "error in (no error)"=w751, "Input"=w752) -> ("error out"=w741:errorcluster)  [unwired: 7 in, 1 out]
      }
      frame #1 {
        # "RECONNECT"
        n297 = case shown="Error" w780 {
          selector: w780 -> [w785 w792]
          tunnel: [w784 w789] -> w778
          tunnel: [w785 w790] -> w779
          tunnel: w781 -> [w784 w786]
          frame No Error {
          }
          frame Error {
            n298 = call <vilib>:"Clear Errors.vi"("error in (no error)"=w792) -> ("error out"=w793:errorcluster)  [unwired: 5 in, 1 out]
            n299 = call <vilib>:"disconnect.vi"("error in (no error)"=w793, "S7 Connection in"=w786) -> ("error out"=w791:errorcluster)  [unwired: 8 in, 1 out]
            n300 = call <vilib>:"Clear Errors.vi"("error in (no error)"=w791) -> ("error out"=w788:errorcluster)  [unwired: 5 in, 1 out]
            n301 = call <vilib>:"connect.vi"("PLC Type"=PLC_Type."S7 200" ("PLC Type 2"), "error in (no error)"=w788) -> ("error out"=w790:errorcluster, "S7 Connection out"=w789:T3)  [unwired: 8 in]
          }
        }
        n302 = Unbundle By Name(w780) -> ("status"=w783:bool)
        n303 = Not(x=w783) -> (.not. x?=w782:bool)
        "PLC 2" <- w782
        n304 = global write "Global 1.vi" "PLC 2"(w782) -> ()
      }
    }
    n305 = call "PADMINI_STOP_ALL.vi"("Enum"=enum16{"Read", "Write"}."Read") -> ("Boolean 2"=w734:bool)  [unwired: 9 in, 1 out]
    n306 = local read "stop"() -> (w733:bool)
    n307 = Or(x=w733, y=w734) -> (x .or. y?=w732:bool)
    n308 = Wait (ms)(milliseconds to wait=u32 50) -> ()  [unwired: 1 out]
  }
  n309 = while {
    shift-right: [w794] -> w35
    shift-left: w48 -> [w804]
    shift-right: [w802] -> w59
    shift-left: w49 -> [w803]
    stop <- w797 stop-if-true
    # "OP 10 AND 20"
    n310 = flat-sequence {
      tunnel: [w806] -> w796
      tunnel: [w805] -> w795
      tunnel: w803 -> [w839]
      tunnel: w804 -> [w856]
      tunnel: [w879] -> w802
      tunnel: [w878] -> w794
      tunnel: w796 -> [w881]
      tunnel: w795 -> [w880]
      frame #0 {
        w821 = u16 12 ("Data Block #")
        w846 = u16 4 ("Data Block #")
        # "NEW CHANGES"
        n311 = global read "DATA LOG.vi" "OP 10 SCAN STATUS"() -> (w838:bool)
        n312 = case shown="True" w838 {
          tunnel: w856 -> [w867 w876]
          tunnel: [w868 w875] -> w855
          tunnel: [w867 w874] -> w853
          tunnel: w839 -> [w868 w871]
          frame False {
          }
          frame True {
            w877 = u16 1  # Data Block #
            n313 = call "PADMINI_AUTO_BARCODE_STATUS.vi"("Enum"=enum16{"Read", "Write"}."Read", "error in (no error)"=w871) -> ("error out"=w870:errorcluster, "O/P"=w872:bool[])  [unwired: 8 in]
            n314 = global write "DATA LOG.vi" "OP 10 SCAN STATUS"(FALSE) -> ()
            n315 = call-poly <vilib>:"write DB.vi"("BOOL input array [byte]"=w872, "error in (no error)"=w870, "Data Block #"=w877, "S7 Connection in"=w876) -> ("error out"=w875:errorcluster, "S7 Connection out"=w874:T3)  [unwired: 4 in, 2 out]
          }
        }
        n316 = call-poly <vilib>:"read DB.vi"("error in (no error)"=w855, "Items # [byte]"=u16 2, "Data Block #"=w846, "S7 Connection in"=w853) -> ("error out"=w854:errorcluster, "BOOL result array  [byte]"=w851:bool[], "S7 Connection out"=w848:T3)  [unwired: 5 in]
        n317 = call "PADMINI_AUTO_CYCLE STATE.vi"("Enum"=enum16{"Read", "Write"}."Write", "error in (no error)"=w854, "Input"=w851) -> ("error out"=w849:errorcluster)  [unwired: 7 in, 1 out]
        n318 = call-poly <vilib>:"read DB.vi"("Item offset [byte]"=u32 2, "error in (no error)"=w849, "items #"=u16 1 ("Items # [byte]"), "Data Block #"=w846, "S7 Connection in"=w848) -> ("error out"=w836:errorcluster, "Int result array"=w834:i16[], "S7 Connection out"=w847:T3)  [unwired: 4 in]
        n319 = call "PADMINI_AUTO_CYCLE VALUE 10.vi"("Enum"=enum16{"Read", "Write"}."Write", "error in (no error)"=w836, "Input"=w834) -> ("error out"=w835:errorcluster)  [unwired: 7 in, 1 out]
        n320 = call-poly <vilib>:"read DB.vi"("Item offset [byte]"=u32 3, "error in (no error)"=w835, "items #"=u16 2 ("Items # [byte]"), "Data Block #"=w846, "S7 Connection in"=w847) -> ("error out"=w842:errorcluster, "STRING result Array"=w843:string[], "S7 Connection out"=w833:T3)  [unwired: 3 in, 1 out]
        n321 = call "PADMINI_AUTO_BARCODE_STRING.vi"("Enum"=enum16{"Read", "Write"}."Write", "error in (no error)"=w842, "Input"=w843) -> ("error out"=w809:errorcluster)  [unwired: 7 in, 1 out]
        n322 = global read "DATA LOG.vi" "OP 20 SCAN STATUS"() -> (w832:bool)
        n323 = call "PADMINI_AUTO_BARCODE_STATUS 20.vi"("Enum"=enum16{"Read", "Write"}."Read", "error in (no error)"=w809) -> ("error out"=w808:errorcluster, "O/P"=w807:bool[])  [unwired: 8 in]
        n324 = case shown="True" w832 {
          tunnel: w833 -> [w858 w862]
          tunnel: [w859 w865] -> w812
          tunnel: [w858 w864] -> w811
          tunnel: w808 -> [w859 w861]
          tunnel: w807 -> [_ w860]
          frame False {
          }
          frame True {
            w866 = u16 2  # Data Block #
            n325 = global write "DATA LOG.vi" "OP 20 SCAN STATUS"(FALSE) -> ()
            n326 = call-poly <vilib>:"write DB.vi"("BOOL input array [byte]"=w860, "error in (no error)"=w861, "Data Block #"=w866, "S7 Connection in"=w862) -> ("error out"=w865:errorcluster, "S7 Connection out"=w864:T3)  [unwired: 4 in, 2 out]
          }
        }
        n327 = call-poly <vilib>:"read DB.vi"("error in (no error)"=w812, "Items # [byte]"=u16 2, "Data Block #"=w821, "S7 Connection in"=w811) -> ("error out"=w814:errorcluster, "BOOL result array  [byte]"=w816:bool[], "S7 Connection out"=w819:T3)  [unwired: 5 in]
        n328 = call "PADMINI_AUTO_CYCLE STATE 20.vi"("Enum"=enum16{"Read", "Write"}."Write", "error in (no error)"=w814, "Input"=w816) -> ("error out"=w818:errorcluster)  [unwired: 7 in, 1 out]
        n329 = call-poly <vilib>:"read DB.vi"("Item offset [byte]"=u32 2, "error in (no error)"=w818, "items #"=u16 4 ("Items # [byte]"), "Data Block #"=w821, "S7 Connection in"=w819) -> ("error out"=w829:errorcluster, "Int result array"=w831:i16[], "S7 Connection out"=w820:T3)  [unwired: 4 in]
        n330 = call "PADMINI_AUTO_CYCLE VALUE 20.vi"("Enum"=enum16{"Read", "Write"}."Write", "error in (no error)"=w829, "Input"=w831) -> ("error out"=w830:errorcluster)  [unwired: 7 in, 1 out]
        n331 = call-poly <vilib>:"read DB.vi"("Item offset [byte]"=u32 6, "error in (no error)"=w830, "items #"=u16 7 ("Items # [byte]"), "Data Block #"=w821, "S7 Connection in"=w820) -> ("error out"=w825:errorcluster, "STRING result Array"=w824:string[], "S7 Connection out"=w806:T3)  [unwired: 3 in, 1 out]
        n332 = call "PADMINI_AUTO_BARCODE_STRING2.vi"("Enum"=enum16{"Read", "Write"}."Write", "error in (no error)"=w825, "Input"=w824) -> ("error out"=w805:errorcluster)  [unwired: 7 in, 1 out]
      }
      frame #1 {
        # "RECONNECT"
        n333 = Unbundle By Name(w880) -> ("status"=w883:bool)
        n334 = case shown="Error" w880 {
          selector: w880 -> [w885 w892]
          tunnel: [w884 w889] -> w878
          tunnel: [w885 w890] -> w879
          tunnel: w881 -> [w884 w886]
          frame No Error {
          }
          frame Error {
            n335 = call <vilib>:"Clear Errors.vi"("error in (no error)"=w892) -> ("error out"=w893:errorcluster)  [unwired: 5 in, 1 out]
            n336 = call <vilib>:"disconnect.vi"("error in (no error)"=w893, "S7 Connection in"=w886) -> ("error out"=w891:errorcluster)  [unwired: 8 in, 1 out]
            n337 = call <vilib>:"Clear Errors.vi"("error in (no error)"=w891) -> ("error out"=w888:errorcluster)  [unwired: 5 in, 1 out]
            n338 = call <vilib>:"connect.vi"("PLC Type"=PLC_Type."S7 200" ("PLC Type 2"), "error in (no error)"=w888) -> ("error out"=w890:errorcluster, "S7 Connection out"=w889:T3)  [unwired: 8 in]
          }
        }
        n339 = Not(x=w883) -> (.not. x?=w882:bool)
        "PLC 1" <- w882
        n340 = global write "Global 1.vi" "PLC 1"(w882) -> ()
      }
    }
    n341 = call "PADMINI_STOP_ALL.vi"("Enum"=enum16{"Read", "Write"}."Read") -> ("Boolean 2"=w799:bool)  [unwired: 9 in, 1 out]
    n342 = Or(x="stop", y=w799) -> (x .or. y?=w797:bool)
    n343 = Wait (ms)(milliseconds to wait=u32 50) -> ()  [unwired: 1 out]
  }
  n344 = call <vilib>:"Clear Errors.vi"("error in (no error)"=w2) -> ("error out"=w4:errorcluster)  [unwired: 5 in, 1 out]
  n345 = call <vilib>:"disconnect.vi"("error in (no error)"=w4, "S7 Connection in"=w3) -> ("error out"=w1:errorcluster)  [unwired: 8 in, 1 out]
  n346 = call <vilib>:"Clear Errors.vi"("error in (no error)"=w59) -> ("error out"=w36:errorcluster)  [unwired: 5 in, 1 out]
  n347 = call <vilib>:"disconnect.vi"("error in (no error)"=w36, "S7 Connection in"=w35) -> ("error out"=w34:errorcluster)  [unwired: 8 in, 1 out]
  n348 = call-dynamic "Shutdown.vi"("error in"=w57, "Modbus master in"=w58) -> ("error out"=w56:errorcluster)  [unwired: 9 in]
  n349 = call-dynamic "Shutdown.vi"("error in"=w55, "Modbus master in"=w54) -> ("error out"=w53:errorcluster)  [unwired: 9 in]
  n350 = Merge Errors(w34, w1, w56, w53) -> (w72:errorcluster)
  n351 = call <vilib>:"Simple Error Handler.vi"("error in (no error)"=w72) -> ("error out"=w71:errorcluster)  [unwired: 4 in, 4 out]
  n352 = call <vilib>:"Clear Errors.vi"("error in (no error)"=w71) -> ("error out"=w70:errorcluster)  [unwired: 5 in, 1 out]
  n353 = invoke class="VI" method="FP.Close"(error in=w70) -> (error out=→"error out":errorcluster)  [unwired: 2 in, 2 out]
